vi "Push_Data_via_Public_Client.vi"(5 "Archive File?":bool[](array[boolean]), 6 "application reference":refnum<vi>, 7 "error in (no error)":errorcluster, 8 "Running on Server?":bool, 10 "Path of Files relative to EnFlo Data Root":path[](array[path])) -> (0 "error out":errorcluster)   [LabVIEW 2012]
uses:
  Anemometry/Anemometry Sub Vis/Globals/Constants_global.vi
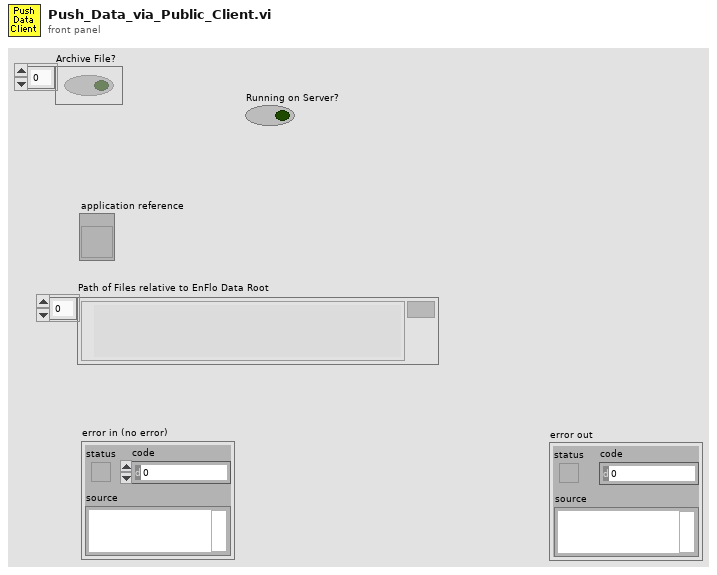
[diagram p1: front panel]
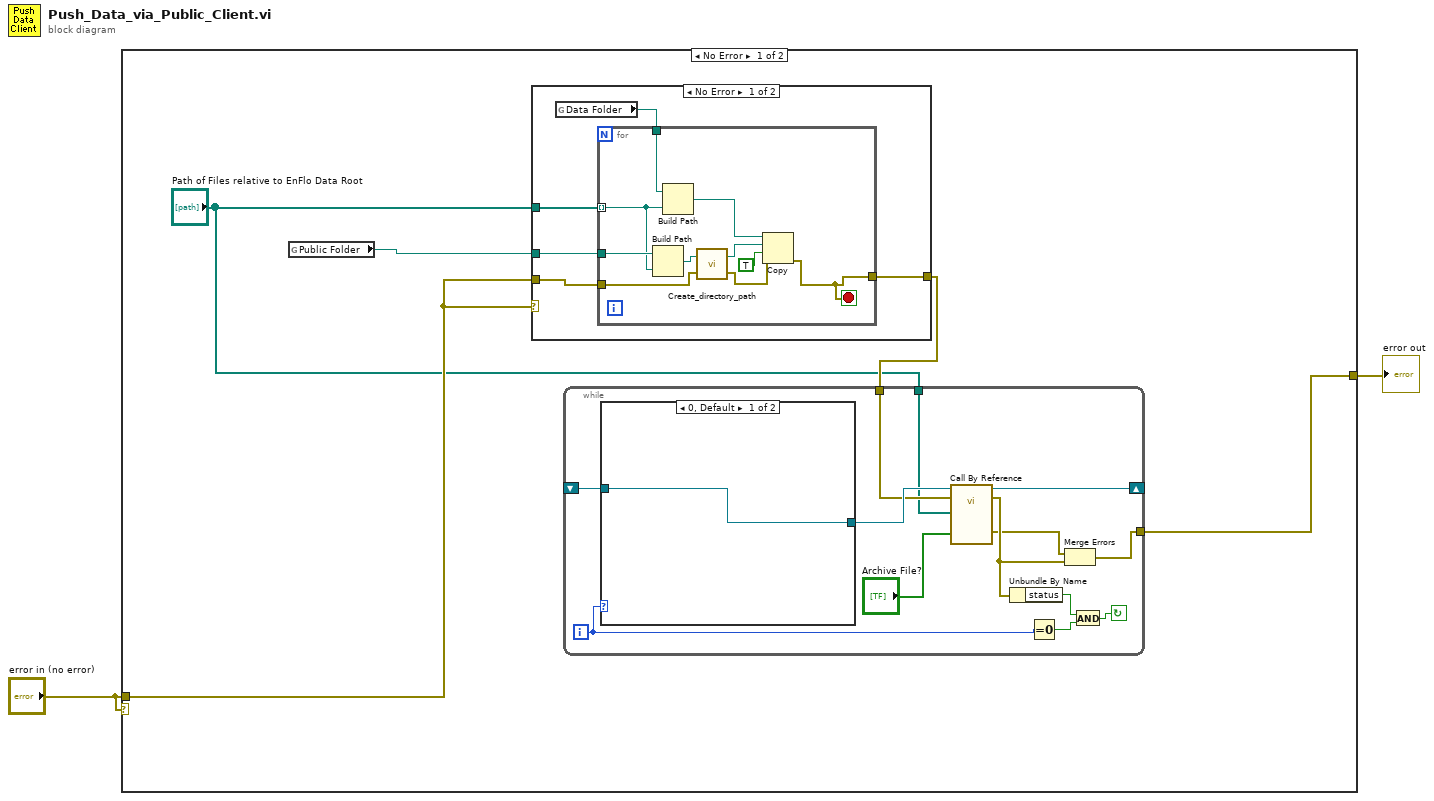
[diagram p0: block diagram]
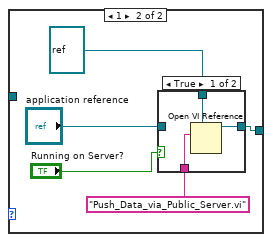
[diagram p2: hidden frame]
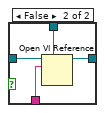
[diagram p3: hidden frame]
diagram:
  n1 = case shown="No Error" "error in (no error)" {
    tunnel: [w5 w50] -> w2
    tunnel: "error in (no error)" -> [w7 w50]
    frame No Error {
      n2 = global read "Constants_global.vi" "Public Folder"() -> (w3:path)
      n3 = case shown="No Error" w7 {
        tunnel: [w34 w49] -> w6
        tunnel: w7 -> [w35 w49]
        tunnel: "Path of Files relative to EnFlo Data Root" -> [w37 _]
        tunnel: w3 -> [w36 _]
        frame No Error {
          n4 = global read "Constants_global.vi" "Data Folder"() -> (w38:path)
          n5 = for {
            tunnel: w38 -> [w40]
            tunnel: w37 -> [w39] mode=indexing
            tunnel: w36 -> [w46]
            tunnel: w35 -> [w42]
            tunnel: [w41] -> w34
            stop <- w41 stop-if-true
            n6 = Build Path(base path=w46, name or relative path=w39) -> (appended path=w47:path)
            n7 = Build Path(base path=w40, name or relative path=w39) -> (appended path=w48:path)
            n8 = call "Create_directory_path.vi"("error in (no error)"=w42, "Path name"=w47) -> ("error out"=w43:errorcluster, "Path name Out"=w45:path)
            n9 = Copy(8:w43, 9:TRUE ("overwrite (F)"), 10:w45, 11:w48) -> (0:w41:errorcluster)  [unwired: 1 in, 2 out]
          }
        }
        frame Error {
        }
      }
      n10 = while {
        shift-right: [w18] -> _
        shift-left: _ -> [w20]
        tunnel: [w8] -> w5
        tunnel: w6 -> [w12]
        tunnel: "Path of Files relative to EnFlo Data Root" -> [w11]
        i -> [w17]
        stop <- w14 continue-if-true
        n11 = case shown="0, Default" w17 {
          tunnel: w20 -> [w21 _]
          tunnel: [w21 w26] -> w19
          frame 0, Default {
          }
          frame 1 {
            n12 = case shown="True" "Running on Server?" {
              tunnel: [w29 w33] -> w26
              tunnel: "application reference" -> [_ w32]
              tunnel: refnum<vi> refnum ("Push Data Server") -> [w28 w31]
              tunnel: "Push_Data_via_Public_Server.vi" -> [w27 w30]
              frame True {
                n13 = Open VI Reference(type specifier VI Refnum (for type only)=w28, vi path=w27) -> (vi reference=w29:refnum<vi>)  [unwired: 2 in, 3 out]
              }
              frame False {
                n14 = Open VI Reference(type specifier VI Refnum (for type only)=w31, application reference (local)=w32, vi path=w30) -> (vi reference=w33:refnum<vi>)  [unwired: 1 in, 3 out]
              }
            }
          }
        }
        n15 = call-by-ref "?"(reference=w19, error in=w12, "Archive File?"="Archive File?", "Path of Files relative to EnFlo Data Root"=w11) -> (reference out=w18:refnum<vi>, error out=w10:errorcluster, "error out"=w9:errorcluster)  [unwired: 2 in]
        n16 = Unbundle By Name(w10) -> ("status"=w15:bool)
        n17 = Equal To 0?(x=w17) -> (x = 0?=w16:bool)
        n18 = Merge Errors(w9, w10) -> (w8:errorcluster)
        n19 = And(x=w15, y=w16) -> (x .and. y?=w14:bool)
      }
    }
    frame Error {
    }
  }
  "error out" <- w2
